vi "Read AI Max.vi"(8 "error in (no error)":errorcluster, 11 "BNT_DAQmx-MCSV in":refnum<class "BNT_DAQmx-MCSV.lvclass">) -> (0 "error out":errorcluster, 2 "AI Max":dbl=5.0, 3 "BNT_DAQmx-MCSV out":refnum<class "BNT_DAQmx-MCSV.lvclass">)   [LabVIEW 2017, in "BNT_DAQmx.lvlib" / "BNT_DAQmx-MCSV.lvclass"]
doc: "Read AI Range Maximum."
uses:
  BNT_DAQmx-MCSV.lvclass
  BNT_DAQmx-MCSV.lvclass/BNT_DAQmx-MCSV.ctl
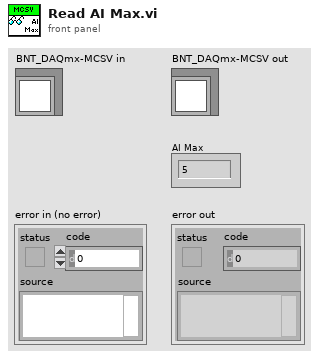
[diagram p1: front panel]
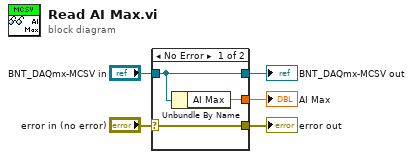
[diagram p0: block diagram]
diagram:
  n1 = case shown="No Error" "error in (no error)" {
    selector: "error in (no error)" -> [w8 w9]
    tunnel: [w8 w9] -> w4
    tunnel: [w7 w10] -> w2
    tunnel: "BNT_DAQmx-MCSV in" -> [w7 w10]
    tunnel: [w6 _] -> w1
    frame No Error {
      n2 = Unbundle By Name(w7) -> ("AI Max"=w6:dbl)
    }
    frame Error {
    }
  }
  "error out" <- w4
  "BNT_DAQmx-MCSV out" <- w2
  "AI Max" <- w1
